vi "workbook new lv.vi"(8 "error in (no error)":errorcluster, 11 "filename":string) -> (0 "error out":errorcluster, 3 "function return":u32)   [LabVIEW 8.6]
doc: "lxw_workbook workbook_new_lv(const char *filename);"
uses:
  pending_lvxlsxwriter/xlsxwriter.dll
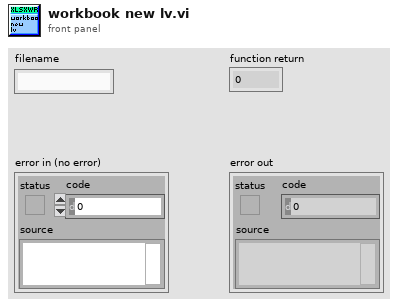
[diagram p1: front panel]
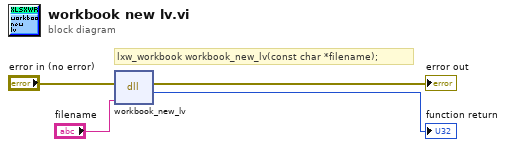
[diagram p0: block diagram]
diagram:
  # "lxw_workbook workbook_new_lv(const char *filename);"
  n1 = dll-call lib="C:/Users/WDAGUtilityAccount/Desktop/pending_lvxlsxwriter/xlsxwriter.*" fn="workbook_new_lv"(error in="error in (no error)", "filename"="filename") -> (error out=→"error out":errorcluster, →"function return":u32)  [unwired: 3 in, 1 out]
